vi "Listbox.vi"(5 "Listbox In":i32(listbox)=3) -> (1 "Numeric":i32, 2 "Listbox Out":i32(listbox)=4)   [LabVIEW 2012]
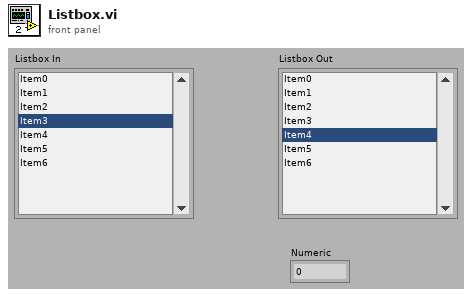
[diagram p1: front panel]
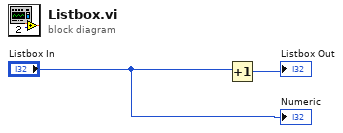
[diagram p0: block diagram]
diagram:
  n1 = Increment(x="Listbox In") -> (x+1=→"Listbox Out":i32)
  "Numeric" <- "Listbox In"
